vi "Image Code Template.vi"() -> ()   [LabVIEW 2012]
uses:
  <vilib>/Rock Robotics/WPI/Camera/WPI_CameraImageSize.ctl
panel:
  out "error out 2":errorcluster
  out "Image Out 3":T1(plugin-control)
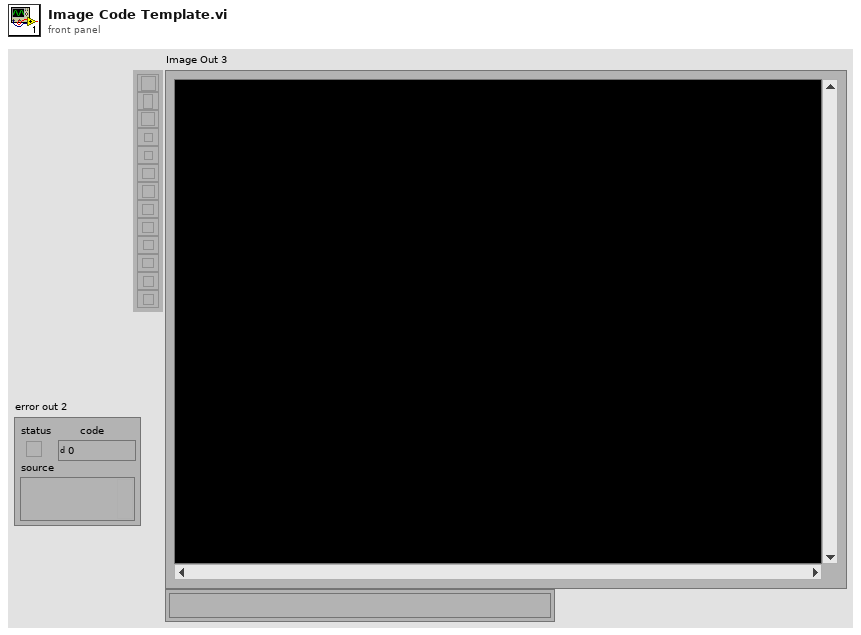
[diagram p1: front panel]
types:
  T1 = typedef "IMAQ Image.ctl" = refnum<image>
  T2 = typedef "Image Type" = u32
  T3 = typedef "WPI_CameraImageSize.ctl" = enum16{"640x480", "320x240", "160x120"}
  T4 = cluster{"fps":i32, "compression":i32, "Image Size":T3}
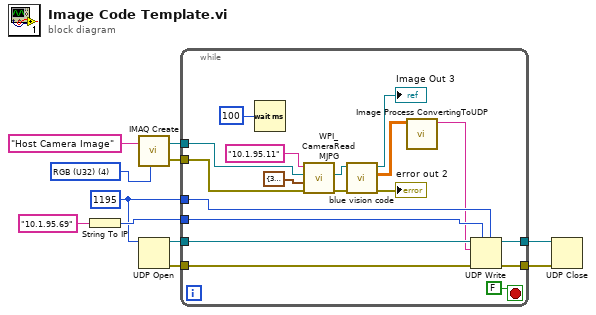
[diagram p0: block diagram]
diagram:
  w1 = u16 1195 ("port")
  w11 = T2 4 items=["Grayscale (U8)", "Grayscale (I16)", "Grayscale (SGL)", "Complex (CSG)", "RGB (U32)", "HSL (U32)", "RGB (U64)"] ("Image Type")
  n1 = String To IP(1:"10.1.95.69" ("name")) -> (0:w2:u32)
  n2 = call "IMAQ Create"("Image Name"="Host Camera Image", "Image Type"=w11) -> ("New Image"=w9:T1, "error out"=w8:errorcluster)  [unwired: 2 in, 1 out]
  n3 = UDP Open(11:w1) -> (port=w6:refnum<k16>, 0:w3:errorcluster)  [unwired: 4 in, 1 out]
  n4 = while {
    tunnel: w9 -> [w28]
    tunnel: w8 -> [w24]
    tunnel: w6 -> [w19]
    tunnel: [w18] -> w5
    tunnel: [w17] -> w4
    tunnel: w3 -> [w16]
    tunnel: w2 -> [w15]
    tunnel: w1 -> [w14]
    stop <- FALSE stop-if-true
    n5 = Wait (ms)(milliseconds to wait=u32 100) -> ()  [unwired: 1 out]
    n6 = call <vilib>:"WPI_CameraRead MJPG.vi"("error in"=w24, "Camera Settings"=T4 {"fps"=30, "compression"=30, "Image Size"=enum."640x480"}, "Image"=w28, "address"="10.1.95.11" ("Robot IP Address")) -> ("error out"=w22:errorcluster, "Image Out"=w23:T1)  [unwired: 5 in, 1 out]
    n7 = call "blue vision code.vi"("error in (no error)"=w22, "Refnum in"=w23) -> ("error out"=→"error out 2":errorcluster, "Particle Measurements (Pixels)"=w13:dbl[][], "Refnum out"=→"Image Out 3":T1)  [unwired: 6 in, 1 out]
    n8 = call "Image Process ConvertingToUDP.vi"("Particle Measurements (Pixels)"=w13) -> ("String"=w12:string)  [unwired: 10 in]
    n9 = UDP Write(address=w15, port or service name=w14, connection ID=w19, data in=w12, 8:w16) -> (error out=w17:errorcluster, 3:w18:refnum<k16>)  [unwired: 1 in]
  }
  n10 = UDP Close(connection ID=w5, 8:w4) -> ()  [unwired: 2 out]
